vi "SaveSpec.vi"(1 "当前量测项目路径":path, 2 "所有量测项目":string[][](table)=[["鱼眼dtX", "-0.100", "0.100", "0.009", "0.009", "1.000000", "0.000000", "96", "1", "0", "-0.250", "0.250"], ["鱼眼dtY", "-0.120", "0.120", "0.009", "0.009", "1.000000", "0.000000", "96", "1", "0", "-0.250", "0.250"]], 3 "其它规格":T3={"其它勾选类规格"={"忽略安全门报警"=FALSE, "忽略光栅报警"=FALSE, "忽略气缸报警"=FALSE, "保存NG图片"=FALSE, "保存OK图片"=FALSE, "保存数据"=FALSE, "实时计算CPK"=FALSE, "良率低于设定值报警"=FALSE, "调试模式每次动态调用后都关闭"=FALSE, "显示更多校验数据"=FALSE, "取消气缸自锁功能"=FALSE}, "其它数据类规格"={"相机像素-毫米换算系数"=15.0, "到第一个拍照点速度"=15.0, "到其它拍照点速度"=0.0, "到待命点速度"=0.0, "到抛料点速度"=0.0, "X轴找原点快速移动距离(mm)"=0.0, "Y轴找原点快速移动距离(mm)"=0.0, "Z轴找原点快速移动距离(mm)"=0.0, "每次到拍照点后延时"=0.0, "良率预警值"=0.0, "生产数量大于多少开始良率预警"=0.0}, "相机名称"="cam1"} {"其它数据类规格"."相机像素-毫米换算系数" format="%.6f"; "其它数据类规格"."到第一个拍照点速度" format="%.4f"}) -> (0 "File out":path)   [LabVIEW 2014]
uses:
  Controls/OtherSpec.ctl
  <vilib>/userdefined/High Color/IMAQdx.ctl
  Global.vi
  <vilib>/Utility/file.llb/Write To Spreadsheet File (string).vi
panel:
  in  "其它数据类规格":T1={"相机像素-毫米换算系数"=15.0, "到第一个拍照点速度"=15.0, "到其它拍照点速度"=0.0, "到待命点速度"=0.0, "到抛料点速度"=0.0, "X轴找原点快速移动距离(mm)"=0.0, "Y轴找原点快速移动距离(mm)"=0.0, "Z轴找原点快速移动距离(mm)"=0.0, "每次到拍照点后延时"=0.0, "良率预警值"=0.0, "生产数量大于多少开始良率预警"=0.0} {"相机像素-毫米换算系数" format="%.6f"; "到第一个拍照点速度" format="%.4f"}
  in  "其它勾选类规格":T2
  out "输出字符串 3":string
  out "输出字符串 2":string
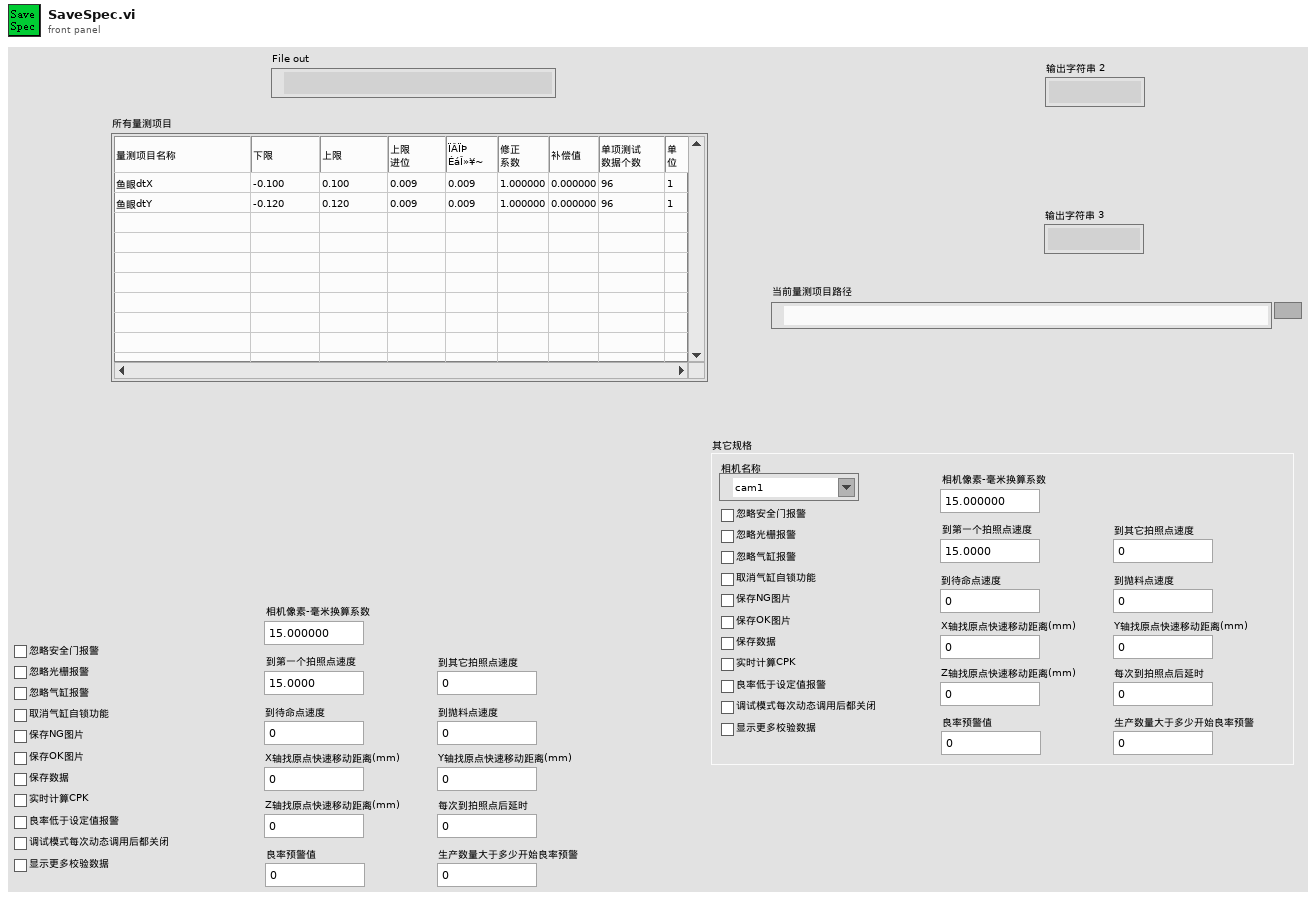
[diagram p1: front panel]
types:
  T1 = typedef "其他数据类规格.ctl" = cluster{"相机像素-毫米换算系数":dbl, "到第一个拍照点速度":dbl, "到其它拍照点速度":dbl, "到待命点速度":dbl, "到抛料点速度":dbl, "X轴找原点快速移动距离(mm)":dbl, "Y轴找原点快速移动距离(mm)":dbl, "Z轴找原点快速移动距离(mm)":dbl, "每次到拍照点后延时":dbl, "良率预警值":dbl, "生产数量大于多少开始良率预警":dbl}
  T2 = typedef "其它勾选类规格.ctl" = cluster{"忽略安全门报警":bool, "忽略光栅报警":bool, "忽略气缸报警":bool, "保存NG图片":bool, "保存OK图片":bool, "保存数据":bool, "实时计算CPK":bool, "良率低于设定值报警":bool, "调试模式每次动态调用后都关闭":bool, "显示更多校验数据":bool, "取消气缸自锁功能":bool}
  T3 = typedef "OtherSpec.ctl" = cluster{"其它勾选类规格":T2, "其它数据类规格":T1, "相机名称":T4}
  T4 = typedef "IMAQdx.ctl" = refnum<k21>
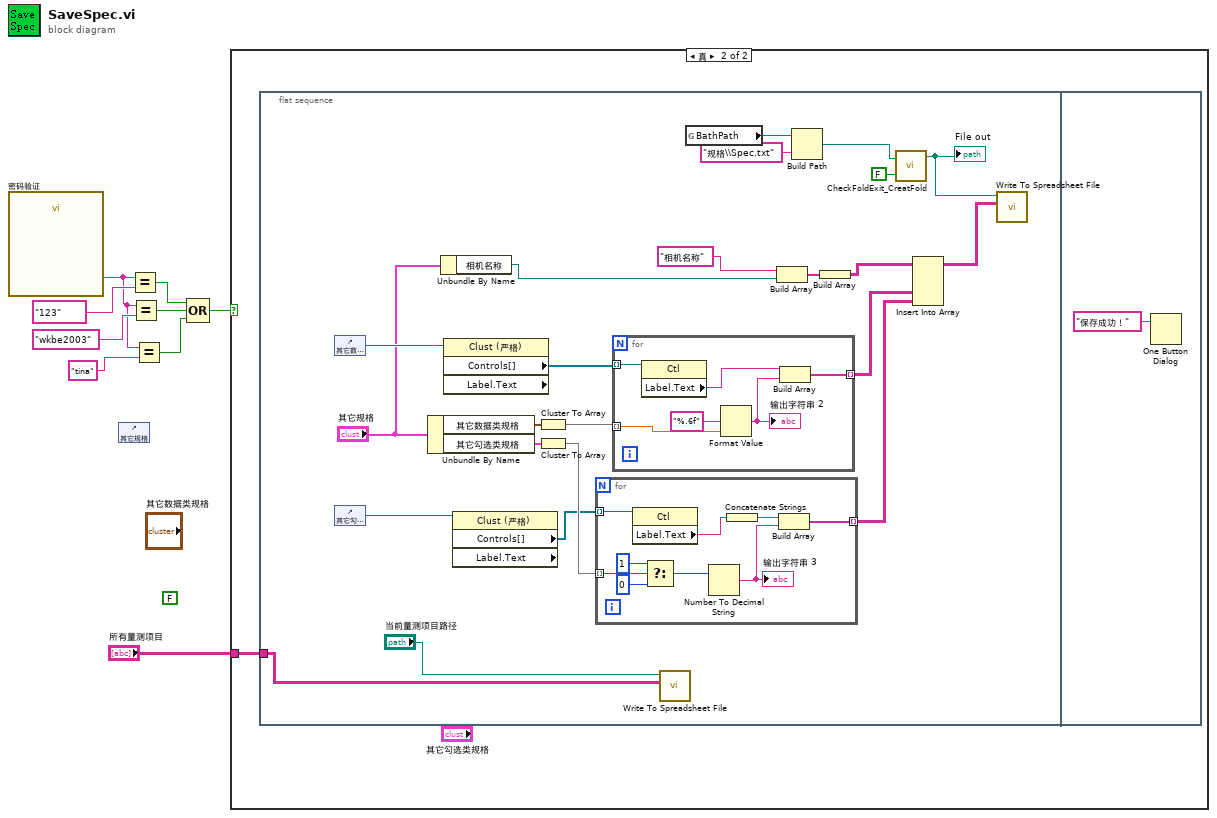
[diagram p0: block diagram]
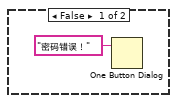
[diagram p2: hidden frame]
diagram:
  (unwired) FALSE ("忽略安全门报警")
  n1 = call "密码验证"() -> ("请输入设置密码"=w3:string)  [unwired: 17 in, 2 out]
  n2 = control-ref of="其它规格"() -> ()  [unwired: 1 out]
  n3 = Equal?(x=w3, y="123") -> (x = y?=w7:bool)
  n4 = Equal?(x=w3, y="wkbe2003") -> (x = y?=w6:bool)
  n5 = Equal?(x=w3, y="tina") -> (x = y?=w4:bool)
  n6 = Compound Arithmetic op=OR(w7, w6, w4) -> (w5:bool)
  n7 = case shown="真" w5 {
    tunnel: "所有量测项目" -> [_ w11]
    frame False {
      n8 = One Button Dialog(message="密码错误！" ("消息")) -> ()  [unwired: 1 in, 1 out]
    }
    frame True {
      n9 = flat-sequence {
        tunnel: w11 -> [w20]
        frame #0 {
          n10 = control-ref of="其它数据类规格"() -> (w21:refnum<vi>)
          n11 = control-ref of="其它勾选类规格"() -> (w24:refnum<vi>)
          n12 = Unbundle By Name("其它规格") -> ("其它数据类规格"=w27:T1, "其它勾选类规格"=w26:T2)
          n13 = Unbundle By Name("其它规格") -> ("相机名称"=w16:T4)
          n14 = property class="Clust (严格)" props=["Controls[]", "Label", "Text"](reference=w21) -> ("Controls[]"=w22:refnum<vi>[])  [unwired: 1 in, 3 out]
          n15 = property class="Clust (严格)" props=["Controls[]", "Label", "Text"](reference=w24) -> ("Controls[]"=w23:refnum<vi>[])  [unwired: 1 in, 3 out]
          n16 = Cluster To Array(cluster=w27) -> (array=w29:dbl[])
          n17 = Cluster To Array(cluster=w26) -> (array=w25:bool[])
          n18 = for {
            tunnel: [w41] -> w12 mode=indexing
            tunnel: w23 -> [w43] mode=indexing
            tunnel: w25 -> [w40] mode=indexing
            n19 = property class="Ctl"(reference=w43) -> ("Label.Text"=w35:string)  [unwired: 1 in, 2 out]
            n20 = Select(t=1, s=w40, f=0 ("t")) -> (s? t:f=w37:i32)
            n21 = Number To Decimal String(number=w37) -> (decimal integer string=w36:string)  [unwired: 1 in]
            "输出字符串 3" <- w36
            n22 = Concatenate Strings(w35) -> (w42:string)
            n23 = Build Array(w42, w36) -> (w41:string[])
          }
          n24 = for {
            tunnel: [w45] -> w13 mode=indexing
            tunnel: w22 -> [w49] mode=indexing
            tunnel: w29 -> [w47] mode=indexing
            n25 = property class="Ctl"(reference=w49) -> ("Label.Text"=w44:string)  [unwired: 1 in, 2 out]
            n26 = Format Value(format string="%.6f" ("format (%.3f)"), value (0)=w47) -> (output string=w46:string)  [unwired: 1 in]
            "输出字符串 2" <- w46
            n27 = Build Array(w44, w46) -> (w45:string[])
          }
          n28 = call-poly <vilib>:"Write To Spreadsheet File.vi"("2D data"=w20, "file path (dialog if empty)"="当前量测项目路径") -> ()  [unwired: 6 in, 1 out]
          n29 = global read "Global.vi" "BathPath"() -> (w32:path)
          n30 = Build Array("相机名称" ("消息"), w16) -> (w15:string[])
          n31 = Build Path(base path=w32, name or relative path="规格\\Spec.txt" ("名称或相对路径")) -> (appended path=w31:path)
          n32 = Build Array(w15) -> (w14:string[][])
          n33 = call "CheckFoldExit_CreatFold.vi"("path in"=w31, "FoldOrFile¡H"=FALSE) -> ("File out"=w33:path)  [unwired: 2 out]
          "File out" <- w33
          n34 = Insert Into Array(array=w14, new element #1=w13, new element #2=w12) -> (w28:string[][])  [unwired: 2 in]
          n35 = call-poly <vilib>:"Write To Spreadsheet File.vi"("2D data"=w28, "file path (dialog if empty)"=w33) -> ()  [unwired: 6 in, 1 out]
        }
        frame #1 {
          n36 = One Button Dialog(message="保存成功！" ("消息")) -> ()  [unwired: 1 in, 1 out]
        }
      }
    }
  }
